vi "set_resonator.vi"(8 "error in (no error)":errorcluster, 10 "resonator":i32=927080) -> (0 "error out":errorcluster, 2 "fundamental (nm)":dbl=536.684118137483 format="%.4f")   [LabVIEW 2017, in "sirah.lvlib"]
uses:
  Sirah_Control_26/Sirah Control Classic 2.6/LabVIEW/Laser/Laser Library LabVIEW 7.1/Stage Reference.ctl
  Sirah_Control_26/Sirah Control Classic 2.6/LabVIEW/Laser/Laser Library LabVIEW 7.1/Laser Position Mode.ctl
  sirah.lvlib
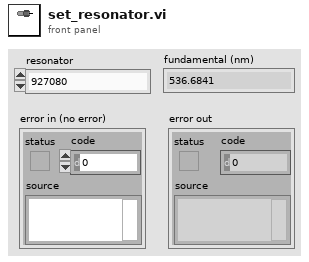
[diagram p1: front panel]
types:
  T1 = typedef "Laser Position Mode.ctl" = enum16{"fundamental, wavelength / nm", "fundamental, wavenumber / cm-1", "fundamental, frequency / GHz", "SHG, wavelength / nm", "SHG, wavenumber /  cm-1", "SHG, frequency / GHz", "DFM @ 1064 nm, wavelength / nm", "DFM @ 1064 nm, wavenumber / cm-1", "DFM @ 1064 nm, freuency / GHz", "OPA @ 1064 nm, wavelength / nm", "OPA @ 1064 nm, wavenumber / cm-1", "OPA @ 1064 nm, frequency / GHz", "THG, wavelength / nm", "THG, wavenumber / cm-1", "THG, frequency / GHz", "SFM @ 1064 nm, wavelength / nm", "SFM @ 1064 nm, wavenumber / cm-1", "SFM @ 1064 nm, frequency / GHz", "SFM @ 532 nm, wavelength / nm", "SFM @ 532 nm, wavenumber / cm-1", "SFM @ 532 nm, frequency / GHz", "SFM @ 355 nm, wavelength / nm", "SFM @ 355 nm, wavenumber / cm-1", "SFM @ 355 nm, frequency / GHz", "SFM @ 266 nm, wavelength / nm", "SFM @ 266 nm, wavenumber / cm-1", "SFM @ 266 nm, frequency / GHz", "NIR, wavelength / nm", "NIR, wavenumber / cm-1", "NIR, frequency / GHz", "DFM @ 355 nm, wavelength / nm", "DFM @ 355 nm, wavenumber / cm-1", "DFM @ 355 nm, frequency / GHz", "MAD @ 1064 nm, wavelength / nm", "MAD @ 1064 nm, wavenumber / cm-1", "MAD @ 1064 nm, frequency / GHz"}
  T2 = enum16{"absolute", "relative", "absolute, quick", "relative, quick"}
  T3 = typedef "Stage Reference.ctl" = enum16{"Resonator", "Conversion(1)", "Conversion(2)", "Conversion(3)", "Conversion(4)", "Conversion(5)", "Conversion(6)", "Conversion(7)"}
  T4 = typedef "Laser Reference.ctl" = refnum<k4>
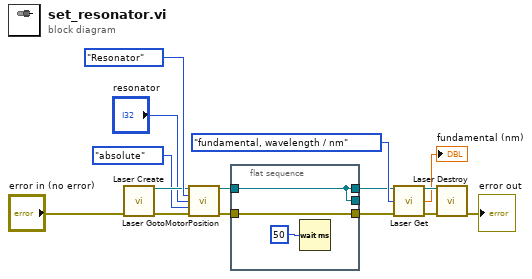
[diagram p0: block diagram]
diagram:
  n1 = call "Laser Create.vi"("error in (no error)"="error in (no error)") -> ("laser out"=w9:T4, "error out"=w7:errorcluster)  [unwired: 13 in]
  n2 = call "Laser GotoMotorPosition.vi"("laser"=w9, "stage ID"=Stage_Reference."Resonator", "position"="resonator", "mode"=T2."absolute", "error in (no error)"=w7) -> ("laser out"=w2:T4, "error out"=w1:errorcluster)  [unwired: 9 in]
  n3 = flat-sequence {
    tunnel: [w18] -> w3
    tunnel: w1 -> [w18]
    tunnel: w2 -> [w16]
    tunnel: [w16] -> _
    tunnel: [w16] -> w4
    frame #0 {
      n4 = Wait (ms)(milliseconds to wait=u32 50) -> ()  [unwired: 1 out]
    }
  }
  n5 = call "Laser Get.vi"("laser"=w4, "laser position mode (fundamental wavelength)"=Laser_Position_Mode."fundamental, wavelength / nm", "error in (no error)"=w3) -> ("laser out"=w15:T4, "position"=→"fundamental (nm)":dbl, "error out"=w13:errorcluster)  [unwired: 10 in]
  n6 = call "Laser Destroy.vi"("laser"=w15, "error in (no error)"=w13) -> ("error out"=→"error out":errorcluster)  [unwired: 13 in]
